vi "FindDevice.vi"(8 "error in (no error)":errorcluster, 11 "KST101 in":refnum<class "KST101.lvclass">) -> (0 "error out":errorcluster, 3 "KST101 out":refnum<class "KST101.lvclass">)   [LabVIEW 2016, in "Stepper Motor Controller.lvlib" / "KST101.lvclass"]
uses:
  KST101.lvclass
  D:/Workspace/ProCyteOne_LaserModuleAlignment/shared/Thorlabs/Kinesis/Dependencies/Thorlabs.MotionControl.DeviceManagerCLI.dll
  Dependencies/Thorlabs.MotionControl.DeviceManagerCLI.dll
  KST101.lvclass/KST101.ctl
  KST-MotorError.ctl
  D:/Workspace/ProCyteOne_LaserModuleAlignment/shared/Thorlabs/Kinesis/Dependencies/Thorlabs.MotionControl.KCube.StepperMotorCLI.dll
  Dependencies/Thorlabs.MotionControl.KCube.StepperMotorCLI.dll
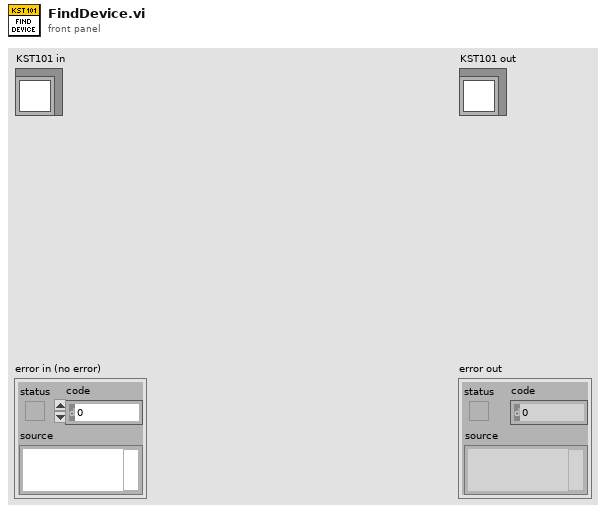
[diagram p1: front panel]
types:
  T1 = typedef "Stepper Motor Controller.lvlib/KST101.lvclass/KST-MotorError.ctl" = enum16{"deviceSerialNotFound"}
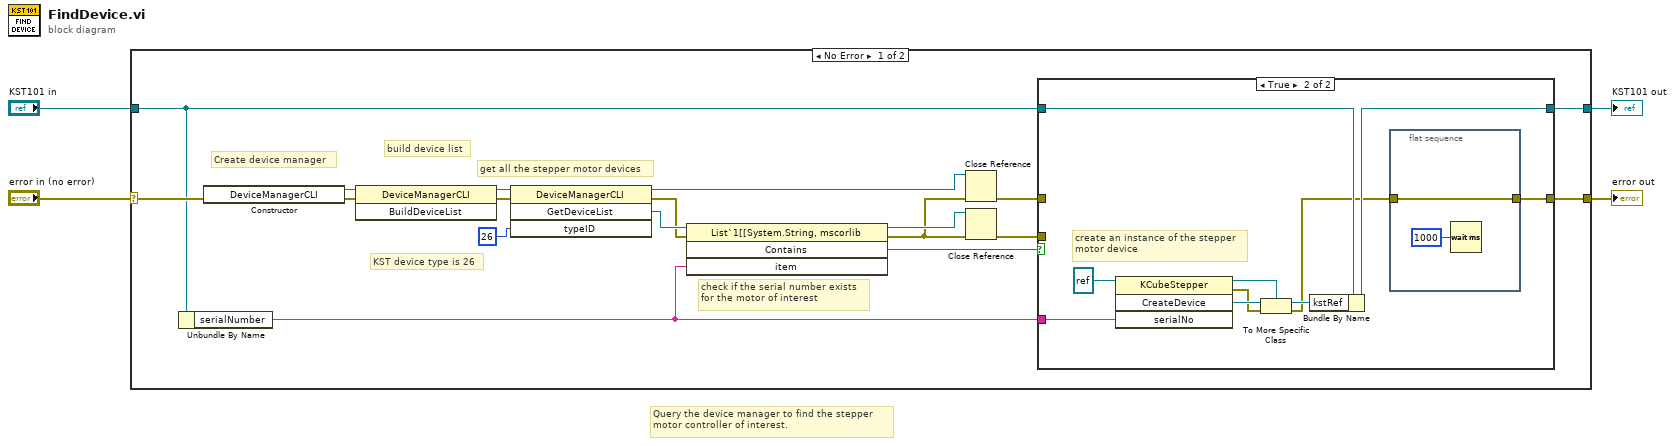
[diagram p0: block diagram]
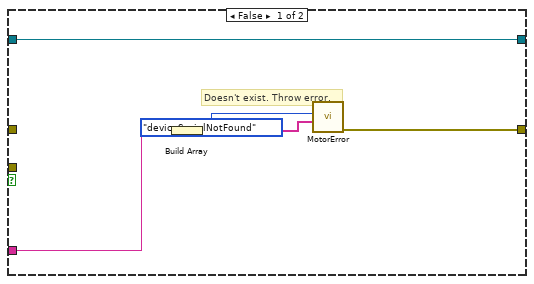
[diagram p2: hidden frame]
diagram:
  # "Query the device manager to find the stepper\nmotor controller of interest."
  n1 = case shown="No Error" "error in (no error)" {
    selector: "error in (no error)" -> [w20 w41]
    tunnel: [w17 w41] -> w3
    tunnel: [w16 w40] -> w1
    tunnel: "KST101 in" -> [w15 w40]
    frame No Error {
      # "KST device type is 26"
      # "check if the serial number exists\nfor the motor of interest"
      # "get all the stepper motor devices"
      # "build device list"
      # "Create device manager"
      n2 = Unbundle By Name(w15) -> ("serialNumber"=w11:string)
      n3 = constructor class="DeviceManagerCLI"(error in=w20) -> (reference out=w22:refnum<k24>, error out=w21:errorcluster)  [unwired: 2 in, 1 out]
      n4 = invoke class="DeviceManagerCLI" method="BuildDeviceList"(reference=w22, error in=w21) -> (reference out=w19:refnum<k24>, error out=w18:errorcluster)  [unwired: 1 in, 1 out]
      n5 = invoke class="DeviceManagerCLI" method="GetDeviceList"(reference=w19, error in=w18, "typeID"=26) -> (reference out=w5:refnum<k24>, error out=w6:errorcluster, "GetDeviceList"=w9:refnum<k24>)  [unwired: 1 in, 1 out]
      n6 = invoke class="List`1[[System.String, mscorlib" method="Contains"(reference=w9, error in=w6, "item"=w11) -> (reference out=w8:refnum<k24>, error out=w7:errorcluster, "Contains"=w12:bool)  [unwired: 1 in, 1 out]
      n7 = Close Reference(reference=w5, error in (no error)=w7) -> (error out=w14:errorcluster)
      n8 = Close Reference(reference=w8, error in (no error)=w7) -> (error out=w13:errorcluster)
      n9 = case shown="True" w12 {
        tunnel: [w23 w29] -> w17
        tunnel: w14 -> [_ _]
        tunnel: w13 -> [_ _]
        tunnel: w11 -> [w25 w37]
        tunnel: [w27 w35] -> w16
        tunnel: w15 -> [w27 w36]
        frame False {
          # "Doesn't exist. Throw error."
          n10 = Build Array(w25) -> (w24:string[])
          n11 = call "MotorError.vi"("args"=w24, "motorErrorType"=KST-MotorError."deviceSerialNotFound") -> ("error out"=w23:errorcluster)  [unwired: 9 in]
        }
        frame True {
          # "create an instance of the stepper\nmotor device"
          n12 = invoke class="KCubeStepper" method="CreateDevice"(reference=refnum<k24> refnum ("GetDeviceList"), "serialNo"=w37) -> (reference out=w33:refnum<k24>, error out=w32:errorcluster, "CreateDevice"=w34:refnum<k24>)  [unwired: 2 in, 1 out]
          n13 = To More Specific Class(target class=w33, reference=w34, error in=w32) -> (specific class reference=w31:refnum<k24>, error out=w30:errorcluster)
          n14 = Bundle By Name(cluster=w36, "kstRef"=w31) -> (w35:refnum<class "KST101.lvclass">)
          n15 = flat-sequence {
            tunnel: [w39] -> w29
            tunnel: w30 -> [w39]
            frame #0 {
              n16 = Wait (ms)(milliseconds to wait=u32 1000) -> ()  [unwired: 1 out]
            }
          }
        }
      }
    }
    frame Error {
    }
  }
  "error out" <- w3
  "KST101 out" <- w1
